vi "Open VI Panel.vi"(8 "error in (no error)":errorcluster, 11 "VI":refnum<vi>) -> (0 "error out":errorcluster)   [LabVIEW 2020, in "UI.lvlib"]
doc: "Open and activate the panel of the specified VI.\n_____\nBased on Delacor QMH Project Template 5.0.0.82."
uses:
  UI.lvlib
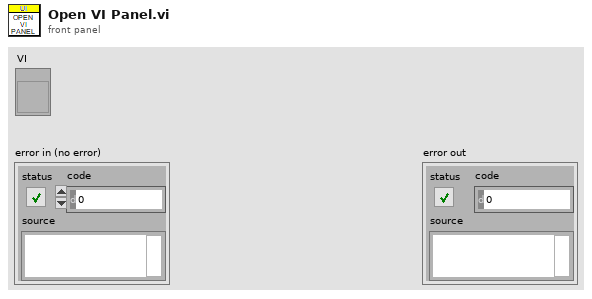
[diagram p1: front panel]
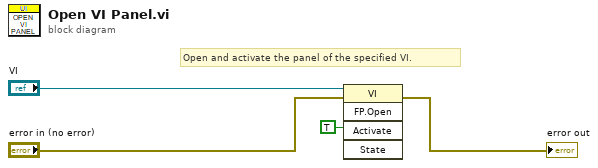
[diagram p0: block diagram]
diagram:
  # "Open and activate the panel of the specified VI."
  n1 = invoke class="VI" method="FP.Open"(reference="VI", error in="error in (no error)", "Activate"=TRUE ("Activate?")) -> (error out=→"error out":errorcluster)  [unwired: 2 in, 4 out]
